vi "建立网络流写入方.vi"(8 "错误输入":errorcluster, 11 "网络流信息":T1={"cRIO名称"="RT", "读取方名称"="2ltITkYLm2nzMX4", "写入方名称 "="zGR2YhZf2vjoZ5U", "网络流大小"=10240, "网络流超时"=5000, "元素类型"={"消息"="", "数据"=variant}}) -> (0 "错误输出":errorcluster, 3 "写入方端点":refnum<k21>)   [LabVIEW 2014]
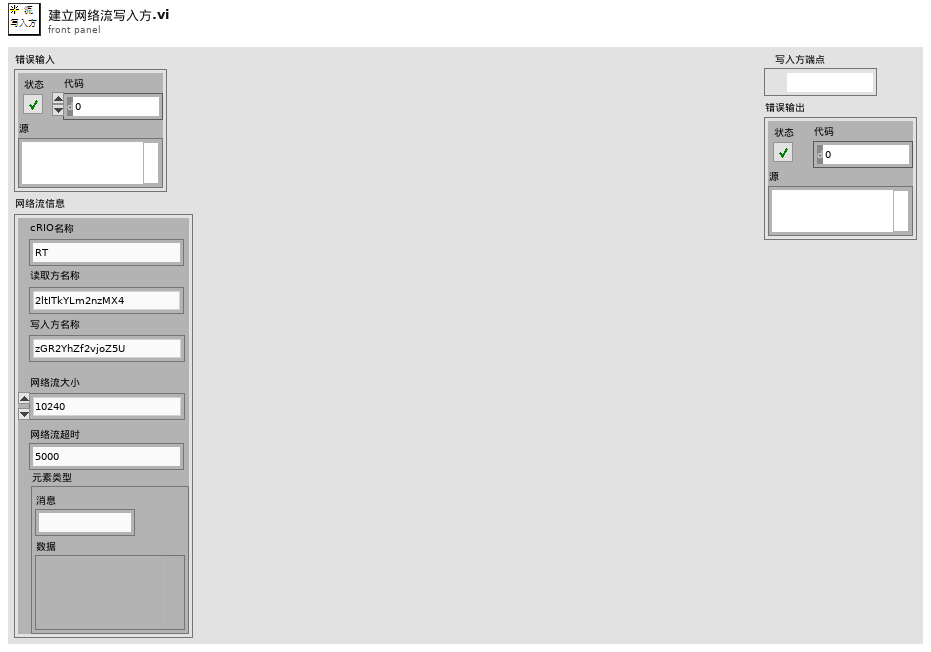
[diagram p1: front panel]
types:
  T1 = cluster{"cRIO名称":string, "读取方名称":string, "写入方名称 ":string, "网络流大小":i32, "网络流超时":i32, "元素类型":cluster{"消息":string, "数据":variant}}
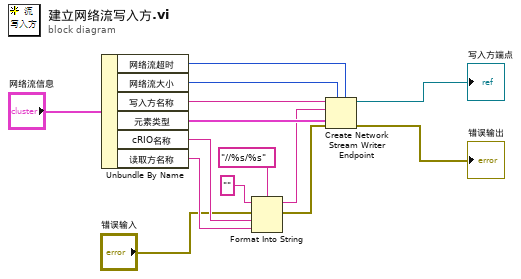
[diagram p0: block diagram]
diagram:
  n1 = Unbundle By Name("网络流信息") -> ("网络流超时"=w10:i32, "网络流大小"=w9:i32, "写入方名称"=w8:string, "元素类型"=w7:cluster{"消息":string, "数据":variant}, "cRIO名称"=w11:string, "读取方名称"=w12:string)
  n2 = Format Into String(format string="//%s/%s" ("格式字符串"), initial string="" ("初始字符串"), error in="错误输入", w11, w12) -> (resulting string=w6:string, error out=w5:errorcluster)
  n3 = Create Network Stream Writer Endpoint(5:w10, 7:w9, 8:w5, 9:w7, 10:w6, 11:w8) -> (0:→"错误输出":errorcluster, 3:→"写入方端点":refnum<k21>)  [unwired: 1 in]
